vi "KGN Set MFC Gase.vi"(7 "mfc Gasnamen in":string[](array[string]), 8 "Fehler (Eingang, kein Fehler)":errorcluster, 9 "Info Cluster":T1, 10 "VISA-Referenz (Eingang)":refnum<visa-resource-name>, 11 "device (Eingang)":u32) -> (0 "Fehler (Ausgang)":errorcluster, 1 "Info Cluster out":T1, 2 "VISA-Referenz (Ausgang)":refnum<visa-resource-name>, 3 "dup device (Ausgang)":u32, 4 "Kommandos gesendet":string)   [LabVIEW 2020, in "Linearisierung v2.lvlib" / "Gasteiler.lvlib" / "HovaCAL_Interface.lvlib" / "KGN.lvlib" / "KGN GUI Set.lvlib"]
uses:
  KGN GUI Set.lvlib
  set/set.lvlib
  Controls/Info Cluster.ctl
  Controls/Controls.lvlib
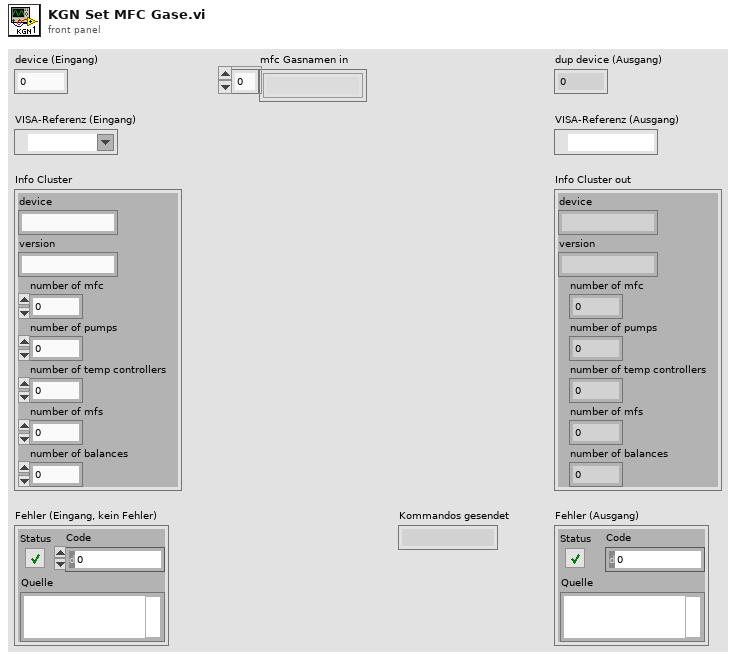
[diagram p1: front panel]
types:
  T1 = typedef "Linearisierung v2.lvlib/Gasteiler.lvlib/HovaCAL_Interface.lvlib/Controls.lvlib/Info Cluster.ctl" = cluster{"device":string, "version":string, "number of mfc":i32, "number of pumps":i32, "number of temp controllers":i32, "number of mfs":i32, "number of balances":i32}
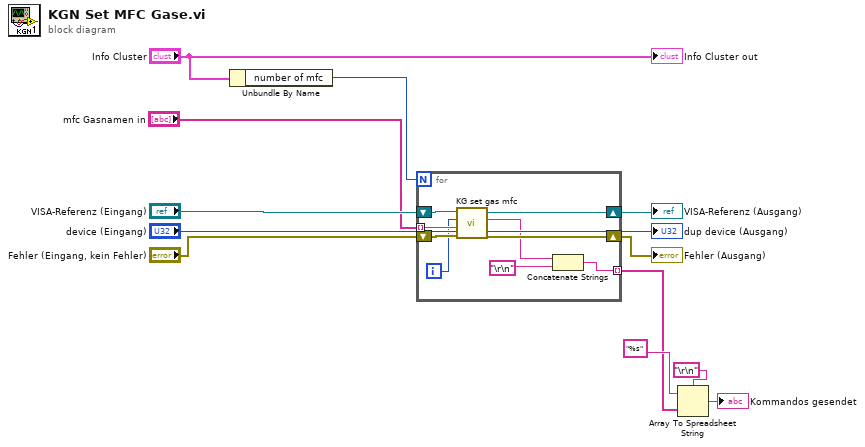
[diagram p0: block diagram]
diagram:
  n1 = Unbundle By Name("Info Cluster") -> ("number of mfc"=w6:i32)
  n2 = for {
    N: w6 -> [_]
    tunnel: "mfc Gasnamen in" -> [w17] mode=indexing
    shift-right: [w18] -> w7
    shift-left: "Fehler (Eingang, kein Fehler)" -> [w21]
    shift-right: [w19] -> w8
    shift-left: "VISA-Referenz (Eingang)" -> [w20]
    tunnel: [w13] -> w2 mode=indexing
    i -> [w16]
    n3 = call "KG set gas mfc.vi"("Fehler (Eingang, kein Fehler)"=w21, "gasname"=w17, "mfc"=w16, "VISA-Ressourcenname"=w20) -> ("Fehler (Ausgang)"=w18:errorcluster, "Kommando gesendet"=w14:string, "VISA-Ressourcenname (Ausgang)"=w19:refnum<visa-resource-name>)  [unwired: 5 in]
    n4 = Concatenate Strings(w14, "\r\n") -> (w13:string)
  }
  "Fehler (Ausgang)" <- w7
  "VISA-Referenz (Ausgang)" <- w8
  n5 = Array To Spreadsheet String(delimiter (Tab)="\r\n", array=w2, 3:"%s" ("Format-String")) -> (spreadsheet string=→"Kommandos gesendet":string)
  "dup device (Ausgang)" <- "device (Eingang)"
  "Info Cluster out" <- "Info Cluster"
